vi "Graveyard - Complex.vi"() -> ()   [LabVIEW 2017]
doc: "A demonstration of using the Graveyard with a slightly more complex refactoring project. This includes step-by-step instructions for each action and one of two methods for displaying the Graveyard."
panel:
  in  "Input":timestamp=timestamp(3614009430.8933406 s since 1904-01-01)
  in  "Stop":bool
  # "Overview: Demonstrates the Graveyard with a more complex refactoring project\nInstructions:\n1. Start the Graveyard using one of the following methods:\n    A. Select View->Bookmark Manager from the menu bar. A dialog will appear. Select \"Graveyard\" from the list and click \"OK\".\n    B. Select Tools->Field R&D Services->Eulogy->Graveyard... \n2. When the Graveyard appears, select \"Main Application Instance\" from the drop down menu on the left, i.e. \"Scope\". The \"Graveyard - Complex\" VI should appear in the tree. Multiple graves and zombies should be listed.\n3. Switch to the block diagram and follow the instructions there to refactor the code"
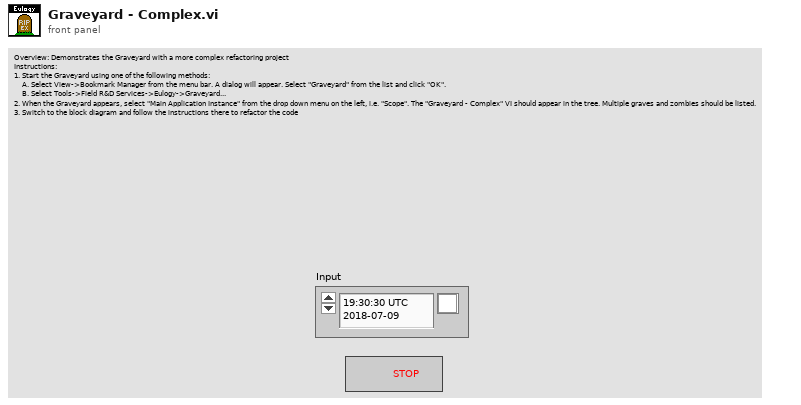
[diagram p1: front panel]
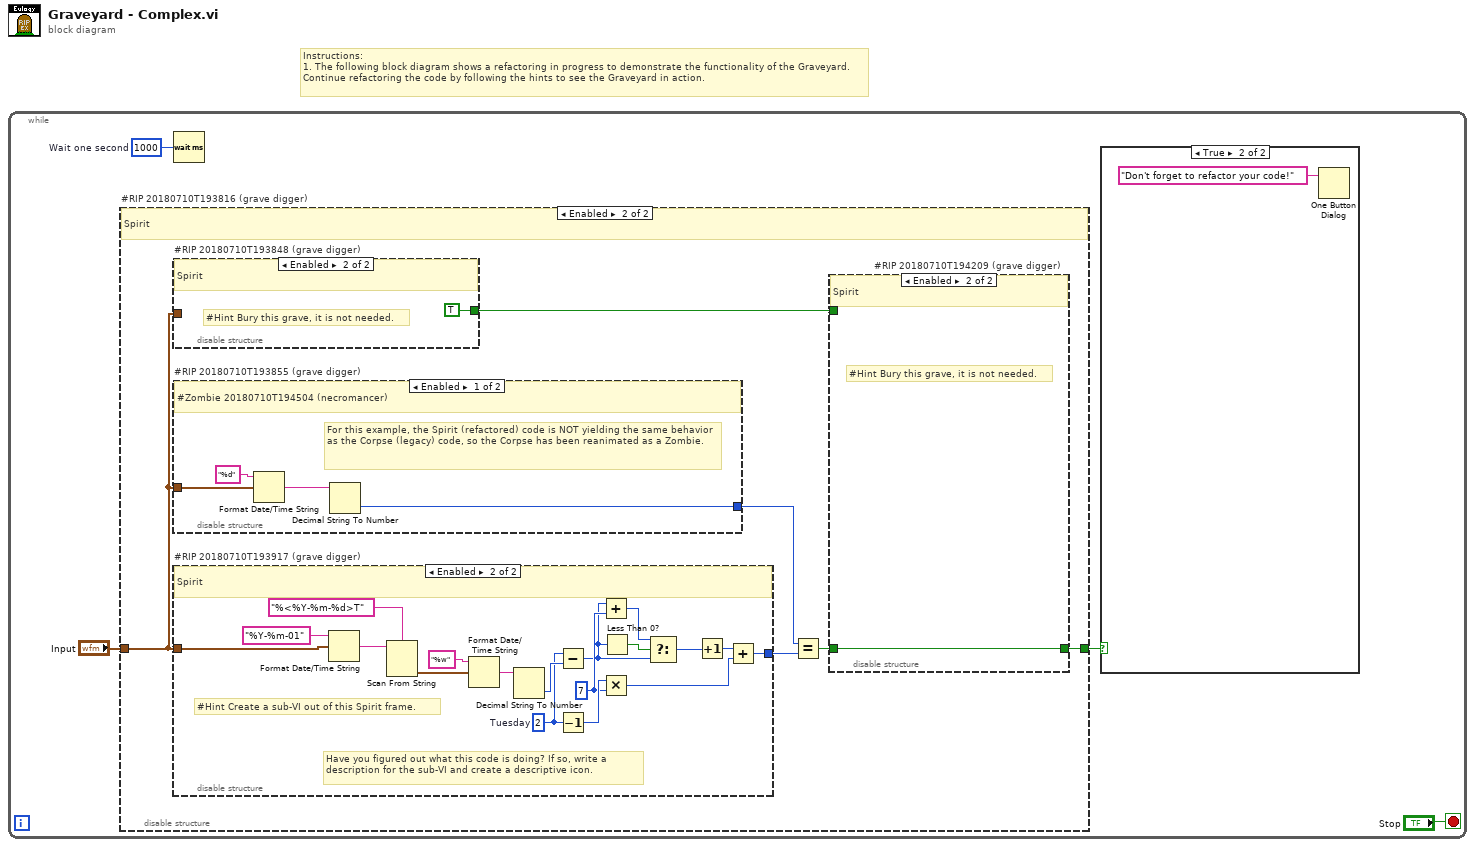
[diagram p0: block diagram]
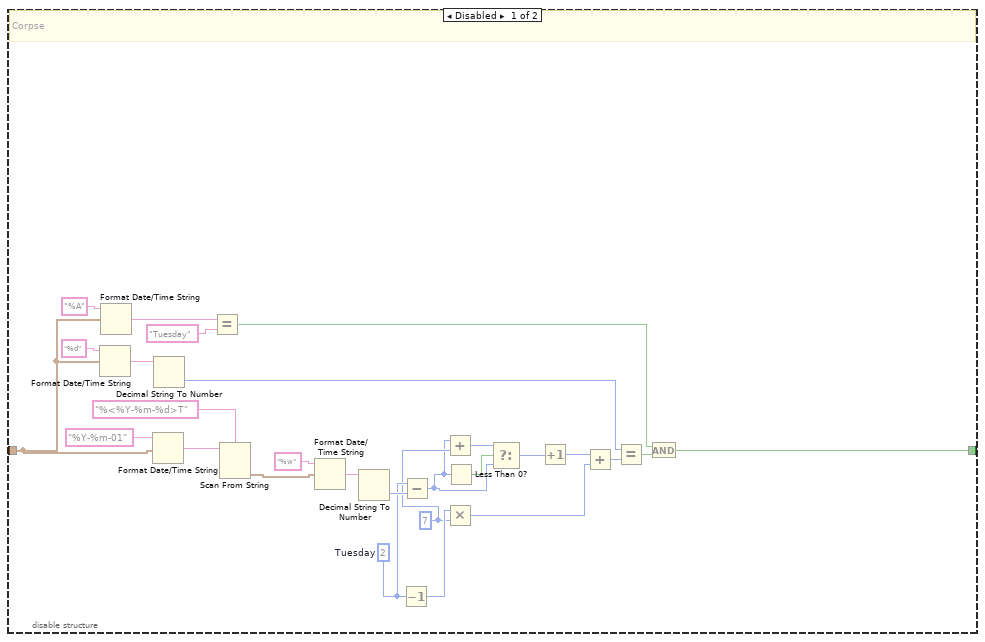
[diagram p2: hidden frame]
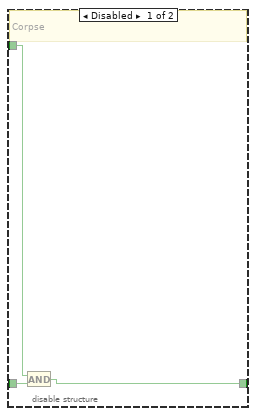
[diagram p3: hidden frame]
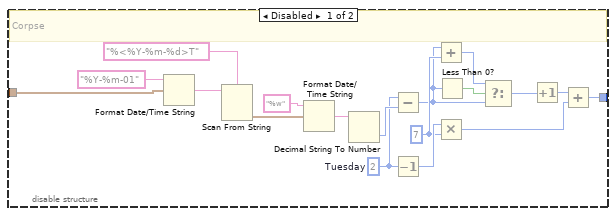
[diagram p4: hidden frame]
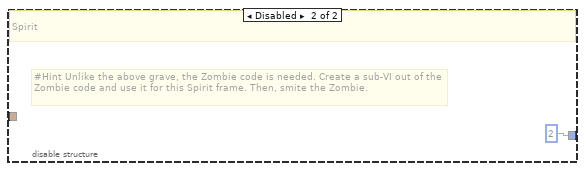
[diagram p5: hidden frame]
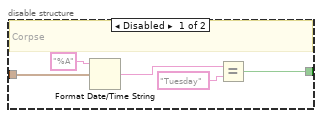
[diagram p6: hidden frame]
diagram:
  # "Instructions:\n1. The following block diagram shows a refactoring in progress to demonstrate the functionality of the Graveyard. Continue refactoring the code by following the hints to see the Graveyard in action."
  n1 = while {
    stop <- "Stop" stop-if-true
    w3 = u32 1000  # Wait one second
    n2 = disable-structure "#RIP 20180710T193816 (grave digger)" shown="Enabled" {
      disable-tunnel: [w6 w33] -> w2
      disable-tunnel: "Input" -> [w5 w32]
      frame Disabled {
        w17 = 7
        w19 = 2  # Tuesday
        # "Corpse"
        n3 = Format Date/Time String(time format string (%c)="%d", seconds (now)=w5) -> (date/time string=w29:string)  [unwired: 1 in]
        n4 = Format Date/Time String(time format string (%c)="%A", seconds (now)=w5) -> (date/time string=w28:string)  [unwired: 1 in]
        n5 = Format Date/Time String(time format string (%c)="%Y-%m-01", seconds (now)=w5) -> (date/time string=w24:string)  [unwired: 1 in]
        n6 = Decimal String To Number(string=w29) -> (number=w8:i32)  [unwired: 2 in, 1 out]
        n7 = Equal?(x=w28, y="Tuesday") -> (x = y?=w10:bool)
        n8 = Scan From String(format string="%<%Y-%m-%d>T", input string=w24) -> (output 1=w23:timestamp)  [unwired: 3 in, 3 out]
        n9 = Format Date/Time String(time format string (%c)="%w", seconds (now)=w23) -> (date/time string=w21:string)  [unwired: 1 in]
        n10 = Decimal String To Number(string=w21) -> (number=w20:i32)  [unwired: 2 in, 1 out]
        n11 = Decrement(x=w19) -> (x-1=w18:i32)
        n12 = Subtract(x=w19, y=w20) -> (x-y=w14:i32)
        n13 = Add(x=w14, y=w17) -> (x+y=w15:i32)
        n14 = Multiply(x=w18, y=w17) -> (x*y=w11:i32)
        n15 = Less Than 0?(x=w14) -> (x < 0?=w16:bool)
        n16 = Select(t=w15, s=w16, f=w14) -> (s? t:f=w13:i32)
        n17 = Increment(x=w13) -> (x+1=w12:i32)
        n18 = Add(x=w12, y=w11) -> (x+y=w9:i32)
        n19 = Equal?(x=w8, y=w9) -> (x = y?=w7:bool)
        n20 = And(x=w10, y=w7) -> (x .and. y?=w6:bool)
      }
      frame Enabled {
        # "Spirit"
        n21 = disable-structure "#RIP 20180710T193848 (grave digger)" shown="Enabled" {
          disable-tunnel: [w84 TRUE] -> w37
          disable-tunnel: w32 -> [w83 _]
          frame Disabled {
            # "Corpse"
            n22 = Format Date/Time String(time format string (%c)="%A", seconds (now)=w83) -> (date/time string=w86:string)  [unwired: 1 in]
            n23 = Equal?(x=w86, y="Tuesday") -> (x = y?=w84:bool)
          }
          frame Enabled {
            # "#Hint Bury this grave, it is not needed."
            # "Spirit"
          }
        }
        n24 = disable-structure "#RIP 20180710T193855 (grave digger)" shown="Enabled" {
          disable-tunnel: [w79 2] -> w35
          disable-tunnel: w32 -> [w78 _]
          frame Enabled {
            # "For this example, the Spirit (refactored) code is NOT yielding the same behavior as the Corpse (legacy) code, so the Corpse has been reanimated as a Zombie."
            # "#Zombie 20180710T194504 (necromancer)"
            n25 = Format Date/Time String(time format string (%c)="%d", seconds (now)=w78) -> (date/time string=w80:string)  [unwired: 1 in]
            n26 = Decimal String To Number(string=w80) -> (number=w79:i32)  [unwired: 2 in, 1 out]
          }
          frame Disabled {
            # "#Hint Unlike the above grave, the Zombie code is needed. Create a sub-VI out of the Zombie code and use it for this Spirit frame. Then, smite the Zombie."
            # "Spirit"
          }
        }
        n27 = disable-structure "#RIP 20180710T193917 (grave digger)" shown="Enabled" {
          disable-tunnel: [w43 w61] -> w36
          disable-tunnel: w32 -> [w42 w60]
          frame Disabled {
            w50 = 7
            w52 = 2  # Tuesday
            # "Corpse"
            n28 = Format Date/Time String(time format string (%c)="%Y-%m-01", seconds (now)=w42) -> (date/time string=w57:string)  [unwired: 1 in]
            n29 = Scan From String(format string="%<%Y-%m-%d>T", input string=w57) -> (output 1=w56:timestamp)  [unwired: 3 in, 3 out]
            n30 = Format Date/Time String(time format string (%c)="%w", seconds (now)=w56) -> (date/time string=w54:string)  [unwired: 1 in]
            n31 = Decimal String To Number(string=w54) -> (number=w53:i32)  [unwired: 2 in, 1 out]
            n32 = Subtract(x=w52, y=w53) -> (x-y=w47:i32)
            n33 = Decrement(x=w52) -> (x-1=w51:i32)
            n34 = Add(x=w47, y=w50) -> (x+y=w48:i32)
            n35 = Multiply(x=w51, y=w50) -> (x*y=w44:i32)
            n36 = Less Than 0?(x=w47) -> (x < 0?=w49:bool)
            n37 = Select(t=w48, s=w49, f=w47) -> (s? t:f=w46:i32)
            n38 = Increment(x=w46) -> (x+1=w45:i32)
            n39 = Add(x=w45, y=w44) -> (x+y=w43:i32)
          }
          frame Enabled {
            w68 = 7
            w70 = 2  # Tuesday
            # "Have you figured out what this code is doing? If so, write a description for the sub-VI and create a descriptive icon."
            # "#Hint Create a sub-VI out of this Spirit frame."
            # "Spirit"
            n40 = Format Date/Time String(time format string (%c)="%Y-%m-01", seconds (now)=w60) -> (date/time string=w75:string)  [unwired: 1 in]
            n41 = Scan From String(format string="%<%Y-%m-%d>T", input string=w75) -> (output 1=w74:timestamp)  [unwired: 3 in, 3 out]
            n42 = Format Date/Time String(time format string (%c)="%w", seconds (now)=w74) -> (date/time string=w72:string)  [unwired: 1 in]
            n43 = Decimal String To Number(string=w72) -> (number=w71:i32)  [unwired: 2 in, 1 out]
            n44 = Subtract(x=w70, y=w71) -> (x-y=w65:i32)
            n45 = Decrement(x=w70) -> (x-1=w69:i32)
            n46 = Add(x=w65, y=w68) -> (x+y=w66:i32)
            n47 = Multiply(x=w69, y=w68) -> (x*y=w62:i32)
            n48 = Less Than 0?(x=w65) -> (x < 0?=w67:bool)
            n49 = Select(t=w66, s=w67, f=w65) -> (s? t:f=w64:i32)
            n50 = Increment(x=w64) -> (x+1=w63:i32)
            n51 = Add(x=w63, y=w62) -> (x+y=w61:i32)
          }
        }
        n52 = Equal?(x=w35, y=w36) -> (x = y?=w34:bool)
        n53 = disable-structure "#RIP 20180710T194209 (grave digger)" shown="Enabled" {
          disable-tunnel: w37 -> [w40 _]
          disable-tunnel: w34 -> [w39 w41]
          disable-tunnel: [w38 w41] -> w33
          frame Disabled {
            # "Corpse"
            n54 = And(x=w40, y=w39) -> (x .and. y?=w38:bool)
          }
          frame Enabled {
            # "#Hint Bury this grave, it is not needed."
            # "Spirit"
          }
        }
      }
    }
    n55 = Wait (ms)(milliseconds to wait=w3) -> ()  [unwired: 1 out]
    n56 = case shown="True" w2 {
      frame False {
      }
      frame True {
        n57 = One Button Dialog(message="Don't forget to refactor your code!") -> ()  [unwired: 1 in, 1 out]
      }
    }
  }
